vi "Enqueue Handle Error Message on Error.vi"(8 "Error In":errorcluster) -> (0 "Error Out":errorcluster)   [LabVIEW 2023, in "QSM - Main.lvlib"]
doc: "This VI enqueues a Handle Error message in the message queue at the front if an error occurred previously for the Queued State Machine template."
uses:
  QSM - Main.lvlib
  Controls/Message Queue Element Position.ctl
  Controls/State Machine Message.ctl
  Enqueue Message (Single).vi
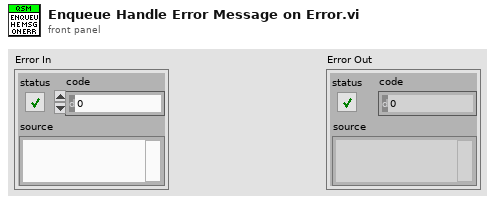
[diagram p1: front panel]
types:
  T1 = typedef "QSM - Main.lvlib/State Machine Message.ctl" = enum16{"Initialize", "Handle Error", "Exit"}
  T2 = typedef "QSM - Main.lvlib/Message Queue Element Position.ctl" = enum16{"Front", "Back"}
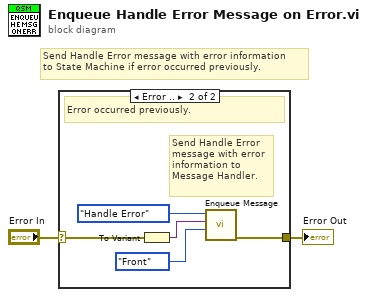
[diagram p0: block diagram]
diagram:
  # "Send Handle Error message with error information\nto State Machine if error occurred previously."
  n1 = case shown="Error .." "Error In" {
    selector: "Error In" -> [w3 w8]
    tunnel: [w3 w5] -> w1
    frame No Error {
      # "Error didn't occur previously."
    }
    frame Error {
      # "Send Handle Error\nmessage with error\ninformation to\nMessage Handler."
      # "Error occurred previously."
      n2 = To Variant(anything=w8) -> (Variant=w7:variant)
      n3 = call-poly "Enqueue Message.vi"("Message Position"=Message_Queue_Element_Position."Front", "Data"=w7, "State Machine Message"=State_Machine_Message."Handle Error") -> ("Error Out"=w5:errorcluster)  [unwired: 8 in]
    }
  }
  "Error Out" <- w1
